vi "Position Set Test.vi"(5 "VI reference":refnum<vi>, 7 "Window Bounds":T1, 8 "error in":errorcluster, 11 "Editor Position in":refnum<class "Editor Position.lvclass">) -> (0 "error out":errorcluster, 3 "Editor Position out":refnum<class "Editor Position.lvclass">)   [LabVIEW 2020, in "Editor Position.lvclass"]
doc: "Tests the basic setting of the position of the VI."
uses:
  Editor Position.lvclass
  Editor Position.lvclass/Editor Position.ctl
  <vilib>/Utility/miscctls.llb/LVRectTypeDef.ctl
  vi.lib/LabVIEW Icon API/lv_icon/lv_icon.lvlib
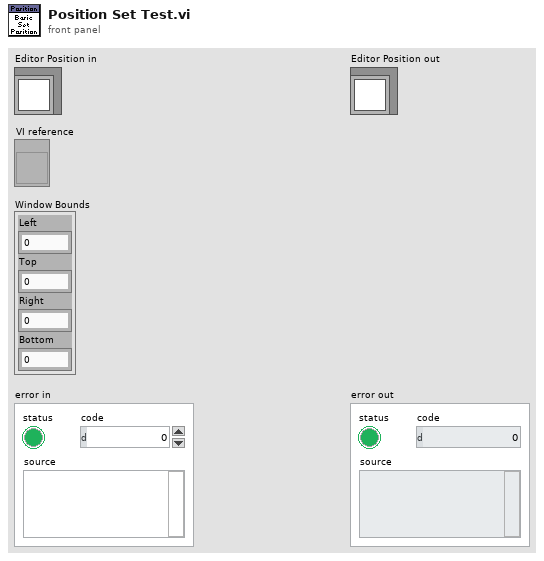
[diagram p1: front panel]
types:
  T1 = typedef "LVRectTypeDef.ctl" = cluster{"Left":i16, "Top":i16, "Right":i16, "Bottom":i16}
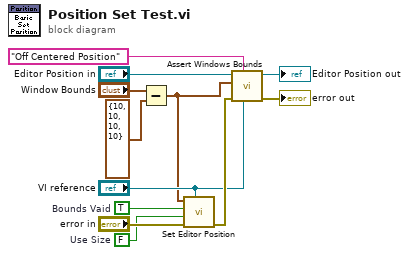
[diagram p0: block diagram]
diagram:
  w8 = FALSE  # Use Size
  w9 = TRUE  # Bounds Vaid
  n1 = Subtract(x="Window Bounds", y=T1 {"Left"=10, "Top"=10, "Right"=10, "Bottom"=10}) -> (x-y=w4:T1)
  n2 = call "Set Editor Position.vi"("IE VI Ref"="VI reference", "error in"="error in", "Use Size"=w8, "Bounds Vaid"=w9, "Window Bounds"=w4) -> ("error out"=w10:errorcluster)  [unwired: 6 in]
  n3 = call "Assert Windows Bounds.vi"("VI reference"="VI reference", "Test Description"="Off Centered Position" ("Description"), "error in"=w10, "Expected Position"=w4, "Editor Position in"="Editor Position in") -> ("error out"=→"error out":errorcluster, "Editor Position out"=→"Editor Position out":refnum<class "Editor Position.lvclass">)  [unwired: 5 in]
